vi "样品标记.vi"(7 "refnum":T1 caption="引用句柄", 10 "测试人员":string, 11 "错误输入（无错误）":errorcluster) -> (2 "样品标记":string[](array[string]), 3 "错误输出":errorcluster, 5 "refnum out":T1 caption="引用句柄输出")   [LabVIEW 2021]
uses:
  <vilib>/Utility/config.llb/Config Data RefNum.ctl
  <vilib>/Utility/config.llb/NI_LVConfig.lvlib
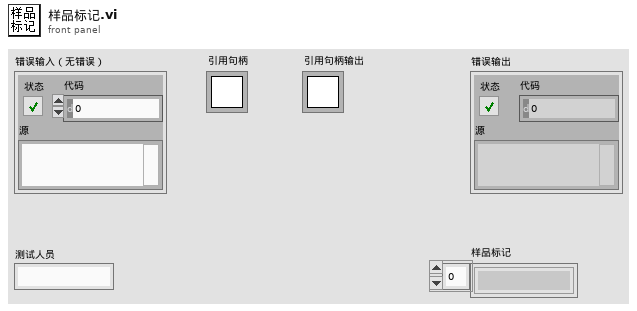
[diagram p1: front panel]
types:
  T1 = typedef "NI_LVConfig.lvlib/Config Data RefNum.ctl" = refnum<k1>
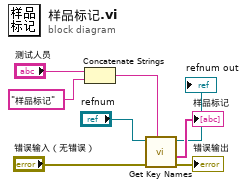
[diagram p0: block diagram]
diagram:
  n1 = Concatenate Strings("测试人员", "样品标记" ("字符串")) -> (w7:string)
  n2 = call <vilib>:"Get Key Names.vi"("section"=w7, "error in (no error)"="错误输入（无错误）", "refnum"="refnum") -> ("error out"=→"错误输出":errorcluster, "key names"=→"样品标记":string[], "refnum out"=→"refnum out":T1)  [unwired: 5 in, 1 out]
